vi "未命名 5.vi"(1 "b":dbl, 2 "x":dbl, 3 "k":dbl) -> (0 "y":dbl)   [LabVIEW 2017]
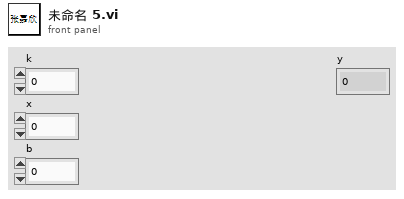
[diagram p1: front panel]
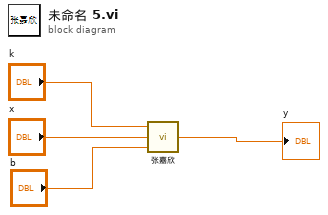
[diagram p0: block diagram]
diagram:
  n1 = call "张嘉欣.vi"("b"="b", "x"="x", "k"="k") -> ("y"=→"y":dbl)
